vi "Spartan HTTP Correct DEV Path.vi"(4 "Normal Path":path) -> (1 "Dev Corrected Path":path)   [LabVIEW 2011]
uses:
  Summitek EXT/OpenG EXT/file/file.llb/Strip Path Extension - String__ogtk.vi
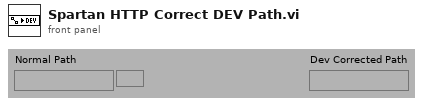
[diagram p1: front panel]
types:
  T1 = enum32{"invalid app kind", "Development System", "Run Time System", "Student Edition", "Embedded LabVIEW", "Evaluation", "Custom"}
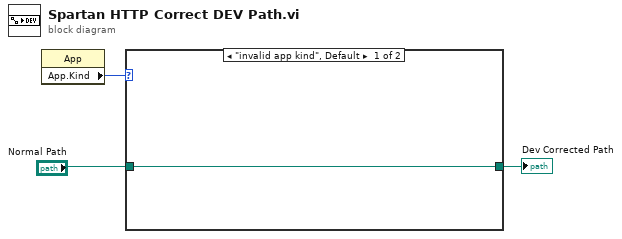
[diagram p0: block diagram]
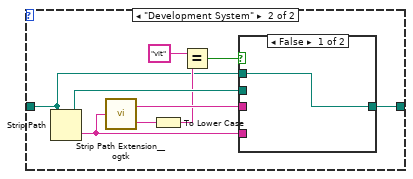
[diagram p2: hidden frame]
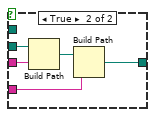
[diagram p3: hidden frame]
diagram:
  n1 = property class="App"() -> ("App.Kind"=w3:T1)  [unwired: 2 in, 2 out]
  n2 = case shown="\"invalid app kind\", Default" w3 {
    tunnel: "Normal Path" -> [w4 w5]
    tunnel: [w4 w10] -> w2
    frame "invalid app kind", Default {
    }
    frame "Development System" {
      n3 = Strip Path(path=w5) -> (stripped path=w12:path, name=w11:string)
      n4 = call-poly "Strip Path Extension__ogtk.vi"("path"=w11) -> ("root"=w13:string, "extension"=w9:string)
      n5 = To Lower Case(string=w9) -> (all lower case string=w8:string)
      n6 = Equal?(x="vit", y=w8) -> (x = y?=w6:bool)
      n7 = case shown="False" w6 {
        tunnel: w13 -> [_ w19]
        tunnel: w12 -> [_ w18]
        tunnel: w11 -> [_ w16]
        tunnel: [w14 w15] -> w10
        tunnel: w5 -> [w14 _]
        frame False {
        }
        frame True {
          n8 = Build Path(base path=w18, name or relative path=w19) -> (appended path=w17:path)
          n9 = Build Path(base path=w17, name or relative path=w16) -> (appended path=w15:path)
        }
      }
    }
  }
  "Dev Corrected Path" <- w2
